vi "Field Draw Robot.vi"(0 "Offset":T17, 1 "picture in":picture, 3 "Draw Number":bool, 5 "Detection Robot":T15 {"height" format="%+4.3f"; "pixel_y" format="%+4.3f"; "pixel_x" format="%+4.3f"; "orientation" format="%+4.3f"; "y" format="%+4.3f"; "confidence" format="%4.3f"; "x" format="%+4.3f"}, 9 "Scale mm/pixel":sgl, 11 "color(black)":u32(colorbox)=16775978, 12 "Robot":T2={"id"=0, "function"=enum."Attacker", "x"=0.0, "y"=0.0, "orientation"=0.0, "v_tangent"=0.0, "v_normal"=0.0, "v_ang"=0.0, "kick_x"=0.0, "kick_z"=0.0, "dribble"=FALSE, "Timestamp"=timestamp(0 s since 1904-01-01), "estimatives"={"est_v_tangent"=0.0, "est_v_normal"=0.0, "est_vx"=0.0, "est_vy"=0.0, "Pos Robot Est"=[]}, "dest_x_kick"=0.0, "dest_y_kick"=0.0, "Gap Coord"=[], "States"=enum."GoToTangent", "Path "=[], "Path  Smooth"=[], "Dest"=[]}, 13 "IA state":T1={"our_robots"=[], "enemy_robots"=[], "balls"=[], "geometry"={"line_width"=0, "field_length"=0, "field_width"=0, "boundary_width"=0, "referee_width"=0, "goal_width"=0, "goal_depth"=0, "goal_wall_width"=0, "center_circle_radius"=0, "defense_radius"=0, "defense_stretch"=0, "free_kick_from_defense_dist"=0, "penalty_spot_from_field_line_dist"=0, "penalty_line_from_spot_dist"=0}, "IA Judge"={"stage"="", "command"="", "our_goalie_id"=0.0, "enemy_goalie_id"=0.0, "command enum"=enum."Halt", "Time"=enum."Azul"}, "Received Timestamp"=timestamp(0 s since 1904-01-01), "Events"={"Touch"=FALSE, "Ball out"=FALSE, "id touch"=0.0, "Ball out of \nVision"=FALSE, "Ball inside \nGoalie area"=FALSE, "Robot not responding"=FALSE, "Robots responding status"=[1.0, 1.0, 1.0, 1.0, 1.0, 1.0], "Enemy Ball \nPossession"=FALSE, "Pass State"=FALSE, "id end of pass"=0.0, "Kick"=FALSE, "Id ini Possession"=0.0, "Ball Possesion"=FALSE, "Id Possesion"=0.0, "Direct Kick"=FALSE}}, 14 "IA Judge.Time":enum16{"Azul", "Amarelo"}(ring), 15 "Draw Targets?":T12) -> (4 "picture out":picture)   [LabVIEW 2017]
uses:
  <vilib>/Utility/miscctls.llb/LVBoundsTypeDef.ctl
  SSL Detection Robot.ctl
  <vilib>/Analysis/Matrix/Datatypes/RealMatrix.ctl
  Core/AI Robot.ctl
  Intel/Functions Enum.ctl
  Intel/AttackerStates.ctl
  Path Planning/RRT/PathDests.ctl
  Path Planning/RRT/PathDest.ctl
  DrawTargets.ctl
  Core/AI Input.ctl
  Core/AI Ball.ctl
  Core/Field Size.ctl
  Core/AI Judge.ctl
  Intel/Command Enum.ctl
  Util/Events/Events.ctl
  <vilib>/Analysis/coordinate.llb/2D Cartesian Coordinate Rotation (Scalar).vi
  <vilib>/Analysis/NI_AALPro.lvlib
  <vilib>/Analysis/Matrix/NI_Matrix.lvlib
panel:
  in  "pen Chute":T13={"Width"=3, "Style"=enum."Solid"}
  in  "pen":T14={"Width"=1.0, "Style"=enum."Solid"}
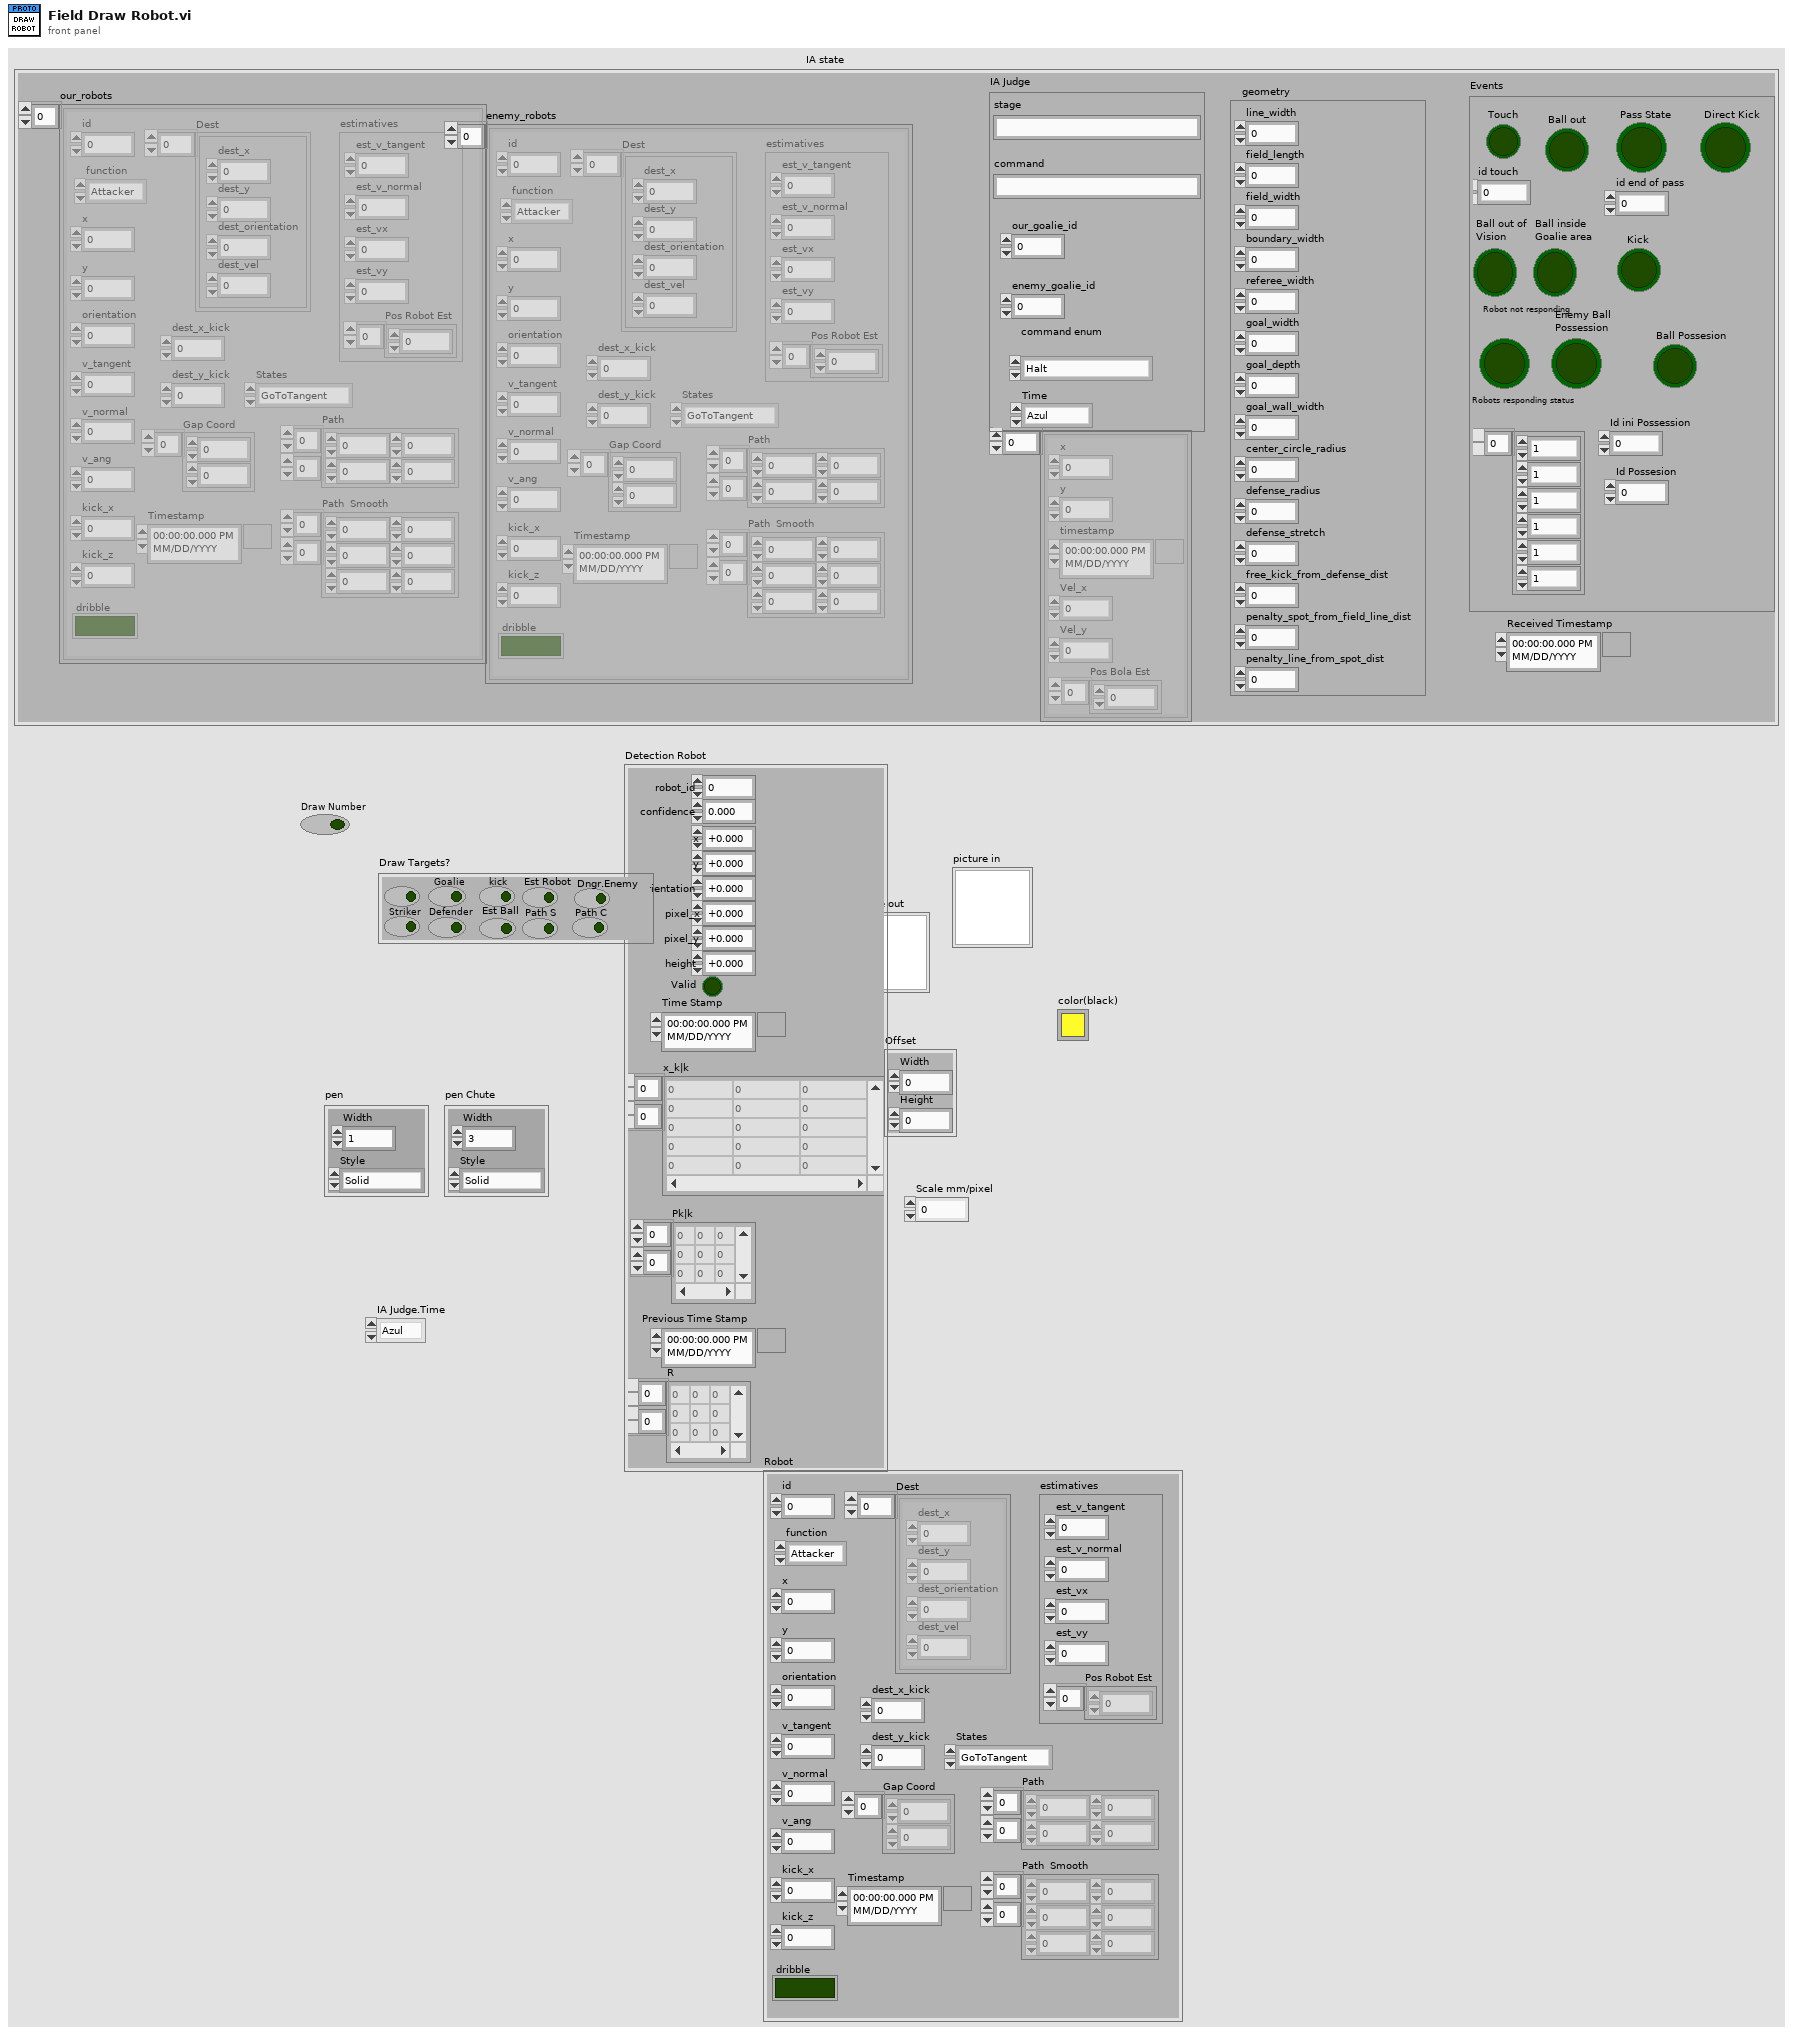
[diagram p1: front panel]
types:
  T1 = typedef "AI Input.ctl" = cluster{"our_robots":T2[], "enemy_robots":T2[], "balls":T7[], "geometry":T8, "IA Judge":T9, "Received Timestamp":timestamp, "Events":T11}
  T2 = typedef "AI Robot.ctl" = cluster{"id":u32, "function":T3, "x":dbl, "y":dbl, "orientation":dbl, "v_tangent":dbl, "v_normal":dbl, "v_ang":dbl, "kick_x":dbl, "kick_z":dbl, "dribble":bool, "Timestamp":timestamp, "estimatives":cluster{"est_v_tangent":dbl, "est_v_normal":dbl, "est_vx":dbl, "est_vy":dbl, "Pos Robot Est":dbl[]}, "dest_x_kick":dbl, "dest_y_kick":dbl, "Gap Coord":dbl[], "States":T4, "Path ":dbl[][], "Path  Smooth":dbl[][], "Dest":T5}
  T3 = typedef "Functions Enum.ctl" = enum16{"Attacker", "Goalie", "Defender", "Striker", "Goto 0", "Dummy", "Kicker", "ZigZag 0", "ZigZag 1", "ZigZag 2", "ZigZag 3", "ZigZag 4", "ZigZag 5", "ZigZag 6", "ZigZag 7", "ZigZag 8", ""}
  T4 = typedef "AttackerStates.ctl" = enum16{"Pass", "GoToTangent", "BallGetting", "GoToKick", ""}
  T5 = typedef "PathDests.ctl" = T6[]
  T6 = typedef "PathDest.ctl" = cluster{"dest_x":dbl, "dest_y":dbl, "dest_orientation":dbl, "dest_vel":dbl}
  T7 = typedef "AI Ball.ctl" = cluster{"x":dbl, "y":dbl, "timestamp":timestamp, "Vel_x":dbl, "Vel_y":dbl, "Pos Bola Est":dbl[]}
  T8 = typedef "Field Size.ctl" = cluster{"line_width":u32, "field_length":u32, "field_width":u32, "boundary_width":u32, "referee_width":u32, "goal_width":u32, "goal_depth":u32, "goal_wall_width":u32, "center_circle_radius":u32, "defense_radius":u32, "defense_stretch":u32, "free_kick_from_defense_dist":u32, "penalty_spot_from_field_line_dist":u32, "penalty_line_from_spot_dist":u32}
  T9 = typedef "AI Judge.ctl" = cluster{"stage":string, "command":string, "our_goalie_id":dbl, "enemy_goalie_id":dbl, "command enum":T10, "Time":enum16{"Azul", "Amarelo"}}
  T10 = typedef "Command Enum.ctl" = enum16{"Halt", "Stop", "Force Start", "PKA Normal Start", "Prepare Kickoff Ally", "PKE Normal Start", "Prepare Kickoff Enemy", "Prepare Penalty Ally", "PPA Normal Start", "Prepare Penalty Enemy", "PPE Normal Start", "Direct Free Enemy", "Direct Free Ally", "Indirect Free Enemy", "Indirect Free Ally", "Timeout Enemy", "Timeout Ally", "Goal Enemy", "Goal Ally", "Ball Placement Enemy", "Ball Placement Ally", "Normal Half Time", "Extra Time Break", "Extra Half Time", "None", "Post Game"}
  T11 = typedef "Events.ctl" = cluster{"Touch":bool, "Ball out":bool, "id touch":dbl, "Ball out of \nVision":bool, "Ball inside \nGoalie area":bool, "Robot not responding":bool, "Robots responding status":dbl[], "Enemy Ball \nPossession":bool, "Pass State":bool, "id end of pass":dbl, "Kick":bool, "Id ini Possession":dbl, "Ball Possesion":bool, "Id Possesion":dbl, "Direct Kick":bool}
  T12 = typedef "DrawTargets.ctl" = cluster{"Attacker":bool, "Striker":bool, "Goalie":bool, "Defender":bool, "kick":bool, "Est Ball":bool, "Est Robot":bool, "Path S":bool, "Path C":bool, "Dngr.Enemy":bool}
  T13 = cluster{"Width":u16, "Style":enum32{"Solid", "Dash", "Dot", "DashDot", "DashDotDot"}}
  T14 = cluster{"Width":dbl, "Style":enum32{"Solid", "Dash", "Dot", "DashDot", "DashDotDot"}}
  T15 = typedef "SSL Detection Robot.ctl" = cluster{"x":sgl, "robot_id":u32, "confidence":sgl, "y":sgl, "orientation":sgl, "pixel_x":sgl, "pixel_y":sgl, "height":sgl, "Valid":bool, "Time Stamp":timestamp, "x_k|k":T16, "Pk|k":T16, "Previous Time Stamp":timestamp, "R":T16}
  T16 = typedef "NI_Matrix.lvlib/RealMatrix.ctl" = dbl[][]
  T17 = typedef "LVBoundsTypeDef.ctl" = cluster{"Width":u32, "Height":u32}
  T18 = cluster{"horizontal":enum16{"left", "center", "right"}, "vertical":enum16{"top", "center", "bottom"}}
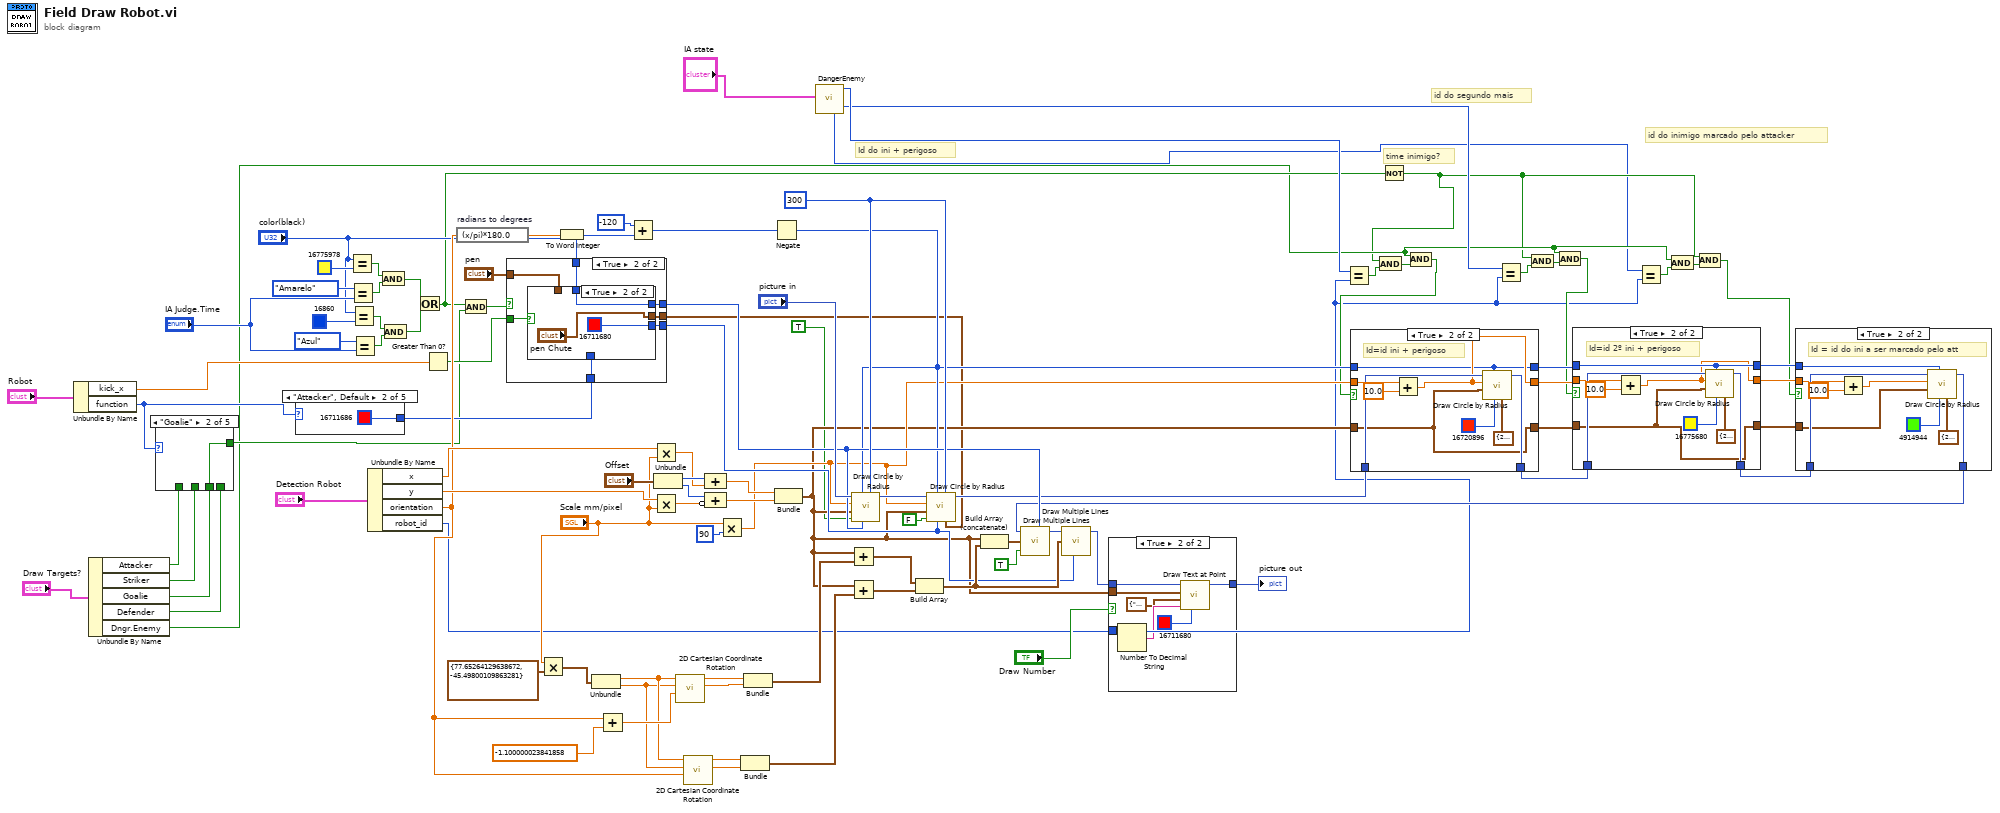
[diagram p0: block diagram]
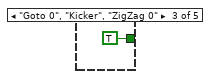
[diagram p6: hidden frame]
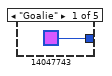
[diagram p11: hidden frame]
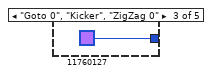
[diagram p12: hidden frame]
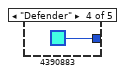
[diagram p13: hidden frame]
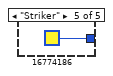
[diagram p14: hidden frame]
diagram:
  w85 = i16 300 ("arc size(360)")
  # "id do inimigo marcado pelo attacker"
  # "id do segundo mais"
  # "time inimigo?"
  # "Id do ini + perigoso"
  n1 = Unbundle By Name("Robot") -> ("kick_x"=w59:dbl, "function"=w35:T3)
  n2 = Unbundle By Name("Draw Targets?") -> ("Attacker"=w41:bool, "Striker"=w40:bool, "Goalie"=w39:bool, "Defender"=w38:bool, "Dngr.Enemy"=w4:bool)
  n3 = case shown="\"Goalie\"" w35 {
    tunnel: [w102 w103 TRUE ("Draw Target Striker?") w105 w106] -> w36
    tunnel: w38 -> [_ _ _ w105 _]
    tunnel: w40 -> [_ _ _ _ w106]
    tunnel: w41 -> [w102 _ _ _ _]
    tunnel: w39 -> [_ w103 _ _ _]
    frame "Attacker", Default {
    }
    frame "Goalie" {
    }
    frame "Goto 0", "Kicker", "ZigZag 0" {
    }
    frame "Defender" {
    }
    frame "Striker" {
    }
  }
  n4 = case shown="\"Attacker\", Default" w35 {
    tunnel: [u32 14047743 ("color(black)") u32 16711686 ("color(black)") u32 11760127 ("color(black)") u32 4390883 ("color(black)") u32 16774186 ("color(black)")] -> w45
    frame "Goalie" {
    }
    frame "Attacker", Default {
    }
    frame "Goto 0", "Kicker", "ZigZag 0" {
    }
    frame "Defender" {
    }
    frame "Striker" {
    }
  }
  n5 = Equal?(x="color(black)", y=u32 16775978 ("color(black)")) -> (x = y?=w52:bool)
  n6 = Equal?(x=enum16{"Azul", "Amarelo"}."Amarelo", y="IA Judge.Time") -> (x = y?=w53:bool)
  n7 = Equal?(x="color(black)", y=u32 16860 ("color(black)")) -> (x = y?=w49:bool)
  n8 = Equal?(x=enum16{"Azul", "Amarelo"}."Azul", y="IA Judge.Time") -> (x = y?=w50:bool)
  n9 = Unbundle By Name("Detection Robot") -> ("x"=w99:sgl, "y"=w100:sgl, "orientation"=w71:sgl, "robot_id"=w5:u32)
  n10 = And(x=w52, y=w53) -> (x .and. y?=w47:bool)
  n11 = And(x=w49, y=w50) -> (x .and. y?=w46:bool)
  n12 = Or(x=w47, y=w46) -> (x .or. y?=w16:bool)
  n13 = Greater Than 0?(x=w59) -> (x > 0?=w44:bool)
  n14 = expression code="(x/pi)*180.0" "radians to degrees"(w71) -> (w89:sgl)
  n15 = And(x=w16, y=w36) -> (x .and. y?=w37:bool)
  n16 = case shown="True" w37 {
    tunnel: [w113 w120] -> w57
    tunnel: [w113 w119] -> w56
    tunnel: "color(black)" -> [w113 w118]
    tunnel: w45 -> [_ w117]
    tunnel: [w112 w116] -> w29
    tunnel: w44 -> [_ w115]
    tunnel: "pen" -> [w112 w114]
    frame False {
    }
    frame True {
      n17 = case shown="True" w115 {
        tunnel: [w122 u32 16711680 ("color(black)")] -> w119
        tunnel: w118 -> [w123 w125]
        tunnel: [w123 w125] -> w120
        tunnel: w117 -> [w122 _]
        tunnel: [w121 "pen Chute"] -> w116
        tunnel: w114 -> [w121 _]
        frame False {
        }
        frame True {
        }
      }
    }
  }
  n18 = Multiply(x="Scale mm/pixel", y=cluster{sgl, sgl} {77.65264, -45.498} ("appended array")) -> (x*y=w66:cluster{sgl, sgl})
  n19 = To Word Integer(number=w89) -> (16bit integer=w88:i16)
  n20 = Unbundle(w66) -> (w73:sgl, w72:sgl)
  n21 = Add(x=w71, y=sgl -1.1 ("theta")) -> (x+y=w74:sgl)
  n22 = Add(x=i16 -120, y=w88) -> (x+y=w87:i16)
  n23 = Multiply(x=w99, y="Scale mm/pixel") -> (x*y=w95:sgl)
  n24 = Multiply(x=w100, y="Scale mm/pixel") -> (x*y=w92:sgl)
  n25 = Unbundle("Offset") -> ("Width"=w96:u32, "Height"=w93:u32)
  n26 = call-poly <vilib>:"2D Cartesian Coordinate Rotation.vi"("theta"=w74, "y"=w72, "x"=w73) -> ("y out"=w76:dbl, "x out"=w77:dbl)  [unwired: 6 in, 1 out]
  n27 = call-poly <vilib>:"2D Cartesian Coordinate Rotation.vi"("theta"=w71, "y"=w72, "x"=w73) -> ("y out"=w69:dbl, "x out"=w70:dbl)  [unwired: 6 in, 1 out]
  n28 = Compound Arithmetic op=ADD(w96, w95) -> (w94:sgl)
  n29 = Compound Arithmetic op=ADD(w93, invert w92) -> (w91:sgl)
  n30 = Multiply(x="Scale mm/pixel", y=i16 90 ("radius")) -> (x*y=w32:sgl)
  n31 = Bundle("x out"=w70, "y out"=w69) -> (w65:cluster{"x out":dbl, "y out":dbl})  [unwired: 1 in]
  n32 = Bundle("x out"=w77, "y out"=w76) -> (w64:cluster{"x out":dbl, "y out":dbl})  [unwired: 1 in]
  n33 = Negate(x=w87) -> (-x=w34:i16)
  n34 = Bundle(w94, w91) -> (w31:cluster{sgl, sgl})  [unwired: 1 in]
  n35 = call "DangerEnemy.vi"("IA Input"="IA state") -> ("id do segundo inimigo\nmais perigoso"=w22:i32, "id do inimigo\nmais perigoso"=w24:u32, "id do inimigo\nmarcado pelo\nStriker"=w1:i32)  [unwired: 5 in, 3 out]
  n36 = Add(x=w31, y=w64) -> (x+y=w62:cluster{dbl, dbl})
  n37 = Add(x=w31, y=w65) -> (x+y=w63:cluster{dbl, dbl})
  n38 = call <vilib>:"Draw Circle by Radius.vi"("arc size(360)"=w85, "color(black)"=w57, "start angle(0)"=w34, "fill?(F)"=TRUE, "pixel center"=w31, "radius"=w32, "picture"="picture in") -> ("new picture"=w60:picture)  [unwired: 4 in]
  n39 = Build Array(w62, w63) -> (w82:cluster{dbl, dbl}[])
  n40 = call <vilib>:"Draw Circle by Radius.vi"("pen"=w29, "arc size(360)"=w85, "color(black)"=w56, "start angle(0)"=w34, "fill?(F)"=FALSE, "pixel center"=w31, "radius"=w32, "picture"=w60) -> ("new picture"=w33:picture)  [unwired: 3 in]
  n41 = Build Array (concatenate)(w31, w82) -> (w80:cluster{dbl, dbl}[])
  n42 = Equal?(x=w24, y=w5) -> (x = y?=w27:bool)
  n43 = Not(x=w16) -> (.not. x?=w3:bool)
  n44 = And(x=w3, y=w27) -> (x .and. y?=w17:bool)
  n45 = And(x=w4, y=w17) -> (x .and. y?=w15:bool)
  n46 = case shown="True" w15 {
    tunnel: w34 -> [w129 w132]
    tunnel: w33 -> [w130 w139]
    tunnel: [w130 w138] -> w21
    tunnel: w32 -> [w128 w137]
    tunnel: w31 -> [w127 w131]
    tunnel: [w129 w132] -> w20
    tunnel: [w128 w133] -> w19
    tunnel: [w127 w131] -> w18
    frame False {
    }
    frame True {
      # "Id=id ini + perigoso"
      n47 = Add(x=w137, y=sgl 10.0) -> (x+y=w133:sgl)
      n48 = call <vilib>:"Draw Circle by Radius.vi"("pen"=T13 {"Width"=2, "Style"=enum."Solid"}, "color(black)"=u32 16720896, "start angle(0)"=w132, "pixel center"=w131, "radius"=w133, "picture"=w139) -> ("new picture"=w138:picture)  [unwired: 5 in]
    }
  }
  n49 = Equal?(x=w22, y=w5) -> (x = y?=w23:bool)
  n50 = And(x=w3, y=w23) -> (x .and. y?=w14:bool)
  n51 = And(x=w4, y=w14) -> (x .and. y?=w13:bool)
  n52 = case shown="True" w13 {
    tunnel: w20 -> [w142 w146]
    tunnel: w21 -> [w143 w152]
    tunnel: [w143 w151] -> w9
    tunnel: w19 -> [w141 w150]
    tunnel: w18 -> [w140 w144]
    tunnel: [w142 w146] -> w12
    tunnel: [w141 w145] -> w11
    tunnel: [w140 w144] -> w10
    frame False {
    }
    frame True {
      # "Id=id 2º ini + perigoso"
      n53 = Add(x=w150, y=sgl 10.0) -> (x+y=w145:sgl)
      n54 = call <vilib>:"Draw Circle by Radius.vi"("pen"=T13 {"Width"=2, "Style"=enum."Solid"}, "color(black)"=u32 16775680, "start angle(0)"=w146, "pixel center"=w144, "radius"=w145, "picture"=w152) -> ("new picture"=w151:picture)  [unwired: 5 in]
    }
  }
  n55 = Equal?(x=w1, y=w5) -> (x = y?=w6:bool)
  n56 = And(x=w4, y=w6) -> (x .and. y?=w7:bool)
  n57 = And(x=w3, y=w7) -> (x .and. y?=w2:bool)
  n58 = case shown="True" w2 {
    tunnel: w12 -> [_ w162]
    tunnel: w9 -> [w153 w161]
    tunnel: [w153 w160] -> w8
    tunnel: w11 -> [_ w159]
    tunnel: w10 -> [_ w158]
    frame False {
    }
    frame True {
      # "Id = id do ini a ser marcado pelo att"
      n59 = Add(x=w159, y=sgl 10.0) -> (x+y=w157:sgl)
      n60 = call <vilib>:"Draw Circle by Radius.vi"("pen"=T13 {"Width"=2, "Style"=enum."Solid"}, "color(black)"=u32 4914944, "start angle(0)"=w162, "pixel center"=w158, "radius"=w157, "picture"=w161) -> ("new picture"=w160:picture)  [unwired: 5 in]
    }
  }
  n61 = call <vilib>:"Draw Multiple Lines.vi"("picture"=w8, "line endpoints"=w80, "fill?(F)"=TRUE, "color(black)"=w57) -> ("new picture"=w81:picture)  [unwired: 5 in]
  n62 = call <vilib>:"Draw Multiple Lines.vi"("picture"=w81, "line endpoints"=w82, "color(black)"=w56) -> ("new picture"=w83:picture)  [unwired: 6 in]
  n63 = case shown="True" "Draw Number" {
    tunnel: [w163 w170] -> w86
    tunnel: w5 -> [_ w168]
    tunnel: w83 -> [w163 w166]
    tunnel: w31 -> [_ w165]
    frame False {
    }
    frame True {
      n64 = Number To Decimal String(number=w168) -> (decimal integer string=w169:string)  [unwired: 1 in]
      n65 = call <vilib>:"Draw Text at Point.vi"("text color(black)"=u32 16711680, "text"=w169, "alignment(left, top)"=T18 {"horizontal"=enum."center", "vertical"=enum."center"}, "origin"=w165, "picture"=w166) -> ("new picture"=w170:picture)  [unwired: 5 in, 1 out]
    }
  }
  "picture out" <- w86
